vi "Cryotel Error decode.vi"(11 "read string array":string[](array[string])) -> (1 "Array 2":i32[](array[numeric]), 2 "Error Code":string, 3 "Error":bool)   [LabVIEW 2019]
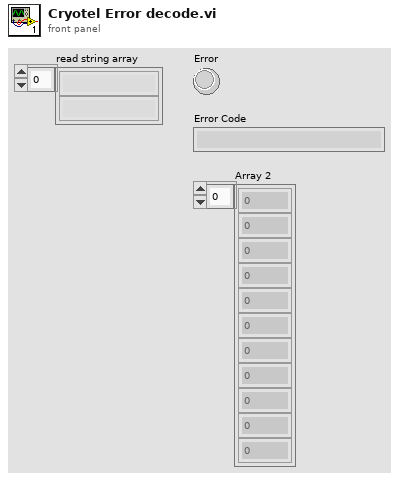
[diagram p1: front panel]
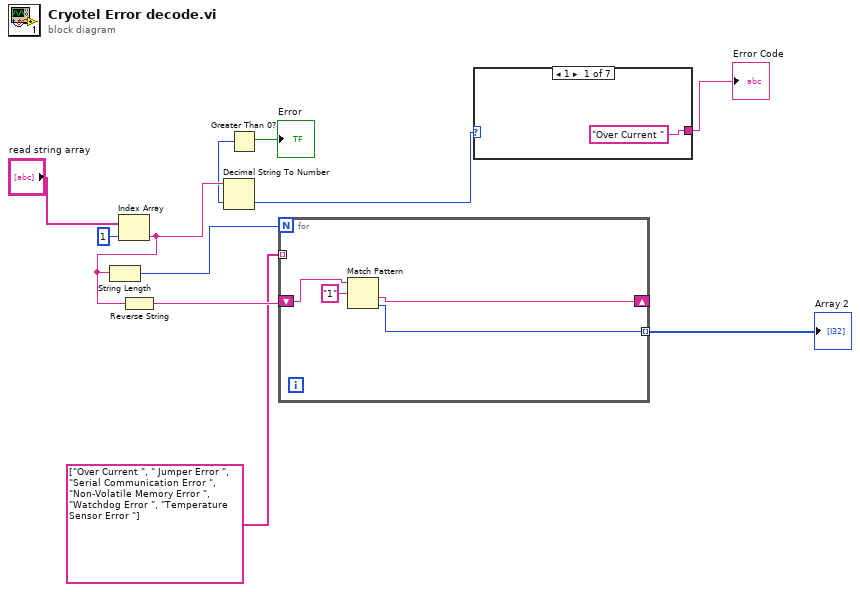
[diagram p0: block diagram]
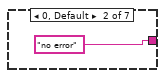
[diagram p2: hidden frame]
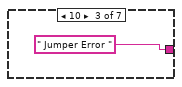
[diagram p3: hidden frame]
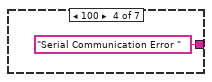
[diagram p4: hidden frame]
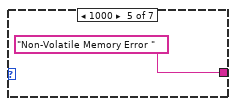
[diagram p5: hidden frame]
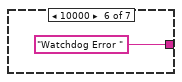
[diagram p6: hidden frame]
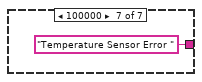
[diagram p7: hidden frame]
diagram:
  n1 = Index Array(array="read string array", index=1) -> (element=w6:string)
  n2 = String Length(string=w6) -> (length=w5:i32)
  n3 = Reverse String(1:w6) -> (0:w8:string)
  n4 = Decimal String To Number(string=w6) -> (number=w3:i32)  [unwired: 2 in, 1 out]
  n5 = Greater Than 0?(x=w3) -> (x > 0?=→"Error":bool)
  n6 = for {
    N: w5 -> [_]
    shift-right: [w13] -> _
    shift-left: w8 -> [w12]
    tunnel: string[] ["Over Current ", " Jumper Error ", "Serial Communication Error ", "Non-Volatile Memory Error ", "Watchdog Error ", "Temperature Sensor Error "] -> [_] mode=indexing
    tunnel: [w11] -> w9 mode=indexing
    n7 = Match Pattern(string=w12, regular expression="1") -> (after substring=w13:string, offset past match=w11:i32)  [unwired: 1 in, 2 out]
  }
  "Array 2" <- w9
  n8 = case shown="1" w3 {
    tunnel: ["Over Current " "no error" " Jumper Error " "Serial Communication Error " "Non-Volatile Memory Error " "Watchdog Error " "Temperature Sensor Error "] -> w10
    frame 1 {
    }
    frame 0, Default {
    }
    frame 10 {
    }
    frame 100 {
    }
    frame 1000 {
    }
    frame 10000 {
    }
    frame 100000 {
    }
  }
  "Error Code" <- w10
